vi "Data Tag Type to DCAF Type.vi"(11 "Data Tag Type":T2) -> (3 "DCAF Data Type":T1)   [LabVIEW 2015, in "SystemLink File configuration.lvclass"]
doc: "Converts Data Tag Type.ctl to the correct DCAF data type. Two data types are required as DCAF does not natively support the Timestamp data type."
uses:
  SystemLink File configuration.lvclass
  Data Tag Type.ctl
  <vilib>/NI/Tag Bus/tag/Data Type.ctl
  <vilib>/NI/Tag Bus/tag/tag descriptor.lvclass
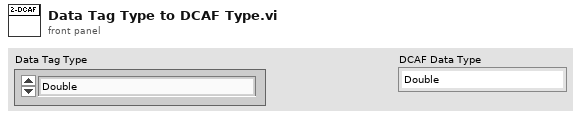
[diagram p1: front panel]
types:
  T1 = typedef "tag bus.lvlib/tag descriptor.lvclass/Data Type.ctl" = enum16{"Double", "Single", "I64", "I32", "I16", "I8", "U64", "U32", "U16", "U8", "Boolean", "String", "Array of Double", "Array of Single", "Array of I64", "Array of I32", "Array of I16", "Array of I8", "Array of U64", "Array of U32", "Array of U16", "Array of U8", "Array of Boolean", "Array of String"}
  T2 = typedef "SystemLink File configuration.lvclass/Data Tag Type.ctl" = enum16{"Double", "Single", "I32", "I16", "I8", "U64", "U32", "U16", "U8", "Boolean", "String", "Timestamp"}
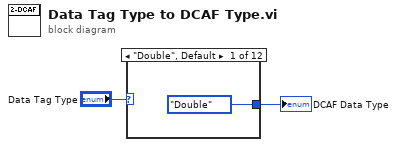
[diagram p0: block diagram]
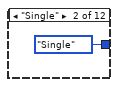
[diagram p2: hidden frame]
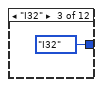
[diagram p3: hidden frame]
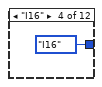
[diagram p4: hidden frame]
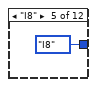
[diagram p5: hidden frame]
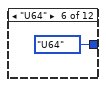
[diagram p6: hidden frame]
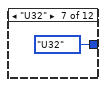
[diagram p7: hidden frame]
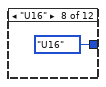
[diagram p8: hidden frame]
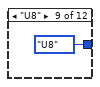
[diagram p9: hidden frame]
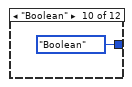
[diagram p10: hidden frame]
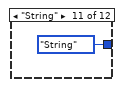
[diagram p11: hidden frame]
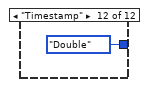
[diagram p12: hidden frame]
diagram:
  n1 = case shown="\"Double\", Default" "Data Tag Type" {
    tunnel: [Data_Type."Double" ("DCAF Data Type") Data_Type."Single" ("DCAF Data Type") Data_Type."I32" ("DCAF Data Type") Data_Type."I16" ("DCAF Data Type") Data_Type."I8" ("DCAF Data Type") Data_Type."U64" ("DCAF Data Type") Data_Type."U32" ("DCAF Data Type") Data_Type."U16" ("DCAF Data Type") Data_Type."U8" ("DCAF Data Type") Data_Type."Boolean" ("DCAF Data Type") Data_Type."String" ("DCAF Data Type") Data_Type."Double" ("DCAF Data Type")] -> w1
    frame "Double", Default {
    }
    frame "Single" {
    }
    frame "I32" {
    }
    frame "I16" {
    }
    frame "I8" {
    }
    frame "U64" {
    }
    frame "U32" {
    }
    frame "U16" {
    }
    frame "U8" {
    }
    frame "Boolean" {
    }
    frame "String" {
    }
    frame "Timestamp" {
    }
  }
  "DCAF Data Type" <- w1
